vi "splitAccelerationData.vi"(8 "ErrorIn":errorcluster, 10 "duration":dbl=1.0 format="%0.2f", 11 "AccelerationDataIn":waveform(dbl)[](array[waveform])) -> (0 "ErrorOut":errorcluster, 2 "AccelerationData-2":waveform(dbl)[](array[waveform]), 3 "AccelerationData-1":waveform(dbl)[](array[waveform]))   [LabVIEW 2019]
uses:
  <vilib>/Waveform/WDTOps.llb/WDT Get Waveform Subset DBL.vi
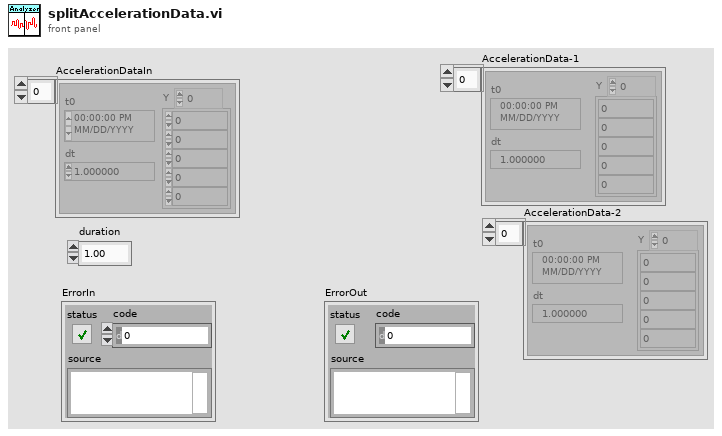
[diagram p1: front panel]
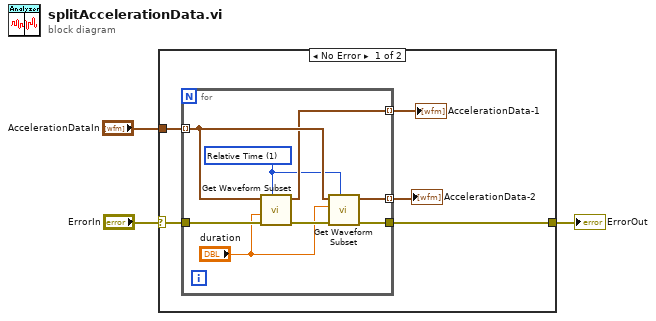
[diagram p0: block diagram]
diagram:
  n1 = case shown="No Error" "ErrorIn" {
    selector: "ErrorIn" -> [w7 w17]
    tunnel: "AccelerationDataIn" -> [w8 _]
    tunnel: [w4 w17] -> w1
    frame No Error {
      n2 = for {
        tunnel: w8 -> [w13] mode=indexing
        tunnel: w7 -> [w16]
        tunnel: [w12] -> w6 mode=indexing
        tunnel: [w11] -> w5 mode=indexing
        tunnel: [w10] -> w4
        w9 = u16 1 items=["Samples", "Relative Time"] ("start/duration format")
        n3 = call-poly <vilib>:"Get Waveform Subset.vi"("start/duration format"=w9, "error in (no error)"=w16, "duration"="duration", "waveform in"=w13) -> ("error out"=w15:errorcluster, "waveform out"=w12:waveform(dbl))  [unwired: 2 in, 2 out]
        n4 = call-poly <vilib>:"Get Waveform Subset.vi"("start/duration format"=w9, "error in (no error)"=w15, "start samples/time"="duration", "waveform in"=w13) -> ("error out"=w10:errorcluster, "waveform out"=w11:waveform(dbl))  [unwired: 2 in, 2 out]
      }
      "AccelerationData-1" <- w6
      "AccelerationData-2" <- w5
    }
    frame Error {
    }
  }
  "ErrorOut" <- w1
